vi "P2_4_Operaciones.vi"() -> ()   [LabVIEW 2020]
panel:
  out "División":string
  out "Multiplicación":string
  out "Resta":string
  out "Suma":string
  in  "No.2":dbl
  in  "No. 1":dbl
  # "Números a utilizar en las operaciones"
  # "Resultados de las operaciones"
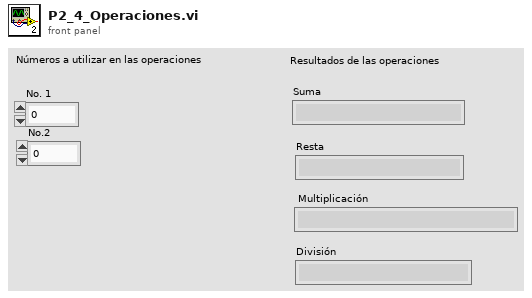
[diagram p1: front panel]
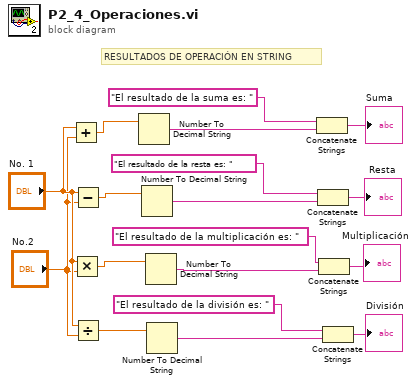
[diagram p0: block diagram]
diagram:
  # "RESULTADOS DE OPERACIÓN EN STRING"
  n1 = Add(x="No. 1", y="No.2") -> (x+y=w16:dbl)
  n2 = Multiply(x="No. 1", y="No.2") -> (x*y=w1:dbl)
  n3 = Subtract(x="No. 1", y="No.2") -> (x-y=w2:dbl)
  n4 = Divide(x="No. 1", y="No.2") -> (x/y=w10:dbl)
  n5 = Number To Decimal String(number=w16) -> (decimal integer string=w14:string)  [unwired: 1 in]
  n6 = Number To Decimal String(number=w2) -> (decimal integer string=w13:string)  [unwired: 1 in]
  n7 = Number To Decimal String(number=w1) -> (decimal integer string=w12:string)  [unwired: 1 in]
  n8 = Number To Decimal String(number=w10) -> (decimal integer string=w11:string)  [unwired: 1 in]
  n9 = Concatenate Strings("El resultado de la suma es: ", w14) -> (→"Suma":string)
  n10 = Concatenate Strings("El resultado de la resta es: ", w13) -> (→"Resta":string)
  n11 = Concatenate Strings("El resultado de la multiplicación es: ", w12) -> (→"Multiplicación":string)
  n12 = Concatenate Strings("El resultado de la división es: ", w11) -> (→"División":string)
